vi "[RT] Finite Acq.vi"() -> ()   [LabVIEW 2025]
doc: "The finite acquisition mode tells the FPGA to acquire a certain number of samples and then terminate the acquisition. In this acquisition mode, the rwfm_ConfigTiming VI calls rwfm_BufferConfig.vi and sets the host application's data buffer size equal to the number of points in the finite acquisition."
uses:
  <vilib>/Utility/error.llb/DialogType.ctl
  <vilib>/NI/cRIO Wfm/ChannelConfig.ctl
  <vilib>/DAQmx/write.llb/DAQmx Write (Analog Wfm 1Chan NSamp).vi
  <vilib>/DAQmx/create/channels.llb/DAQmx Create Channel (AO-Voltage-Basic).vi
  <vilib>/DAQmx/configure/timing.llb/DAQmx Timing (Sample Clock).vi
  <vilib>/DAQmx/miscellaneous.llb/DAQmx Fill In Error Info.vi
  <vilib>/FPGAPlugInAG/cRIO-9045/niLvFpga_Open_cRIO-9045.vi
  <vilib>/rvi/interface/common/dynamic/niFpgaDynamicAddResources.vi
  <vilib>/NI/cRIO Wfm/AcqRead(Wfm).vi
  <vilib>/FPGAPlugInAG/Dynamic/niLvFpga_Close_Dynamic.vi
  <vilib>/rvi/interface/nirviOpenFPGA/nirviOpenFPGA.xnode
  FPGA Bitfiles/criowaveformexam_FPGATarget2_[FPGA]DeltaSigan_kh7RgRjxIrM.lvbitx
  <vilib>/rvi/interface/nirviCloseFPGA/nirviCloseFPGA.xnode
  <vilib>/NI/cRIO Wfm/cRIO Wfm.lvlib
  <resource>/objmgr/daqmx.rc
  <vilib>/measure/NI_MABase.lvlib
panel:
  out "error out":errorcluster
  out "AO Waveform Graph":waveform(dbl)(graph)
  out "Actual AO Sample Rate":dbl=1000.0 format="%0.2f"
  in  "Stop":bool
  out "Acquired Data Graph":waveform(sgl)[](graph)
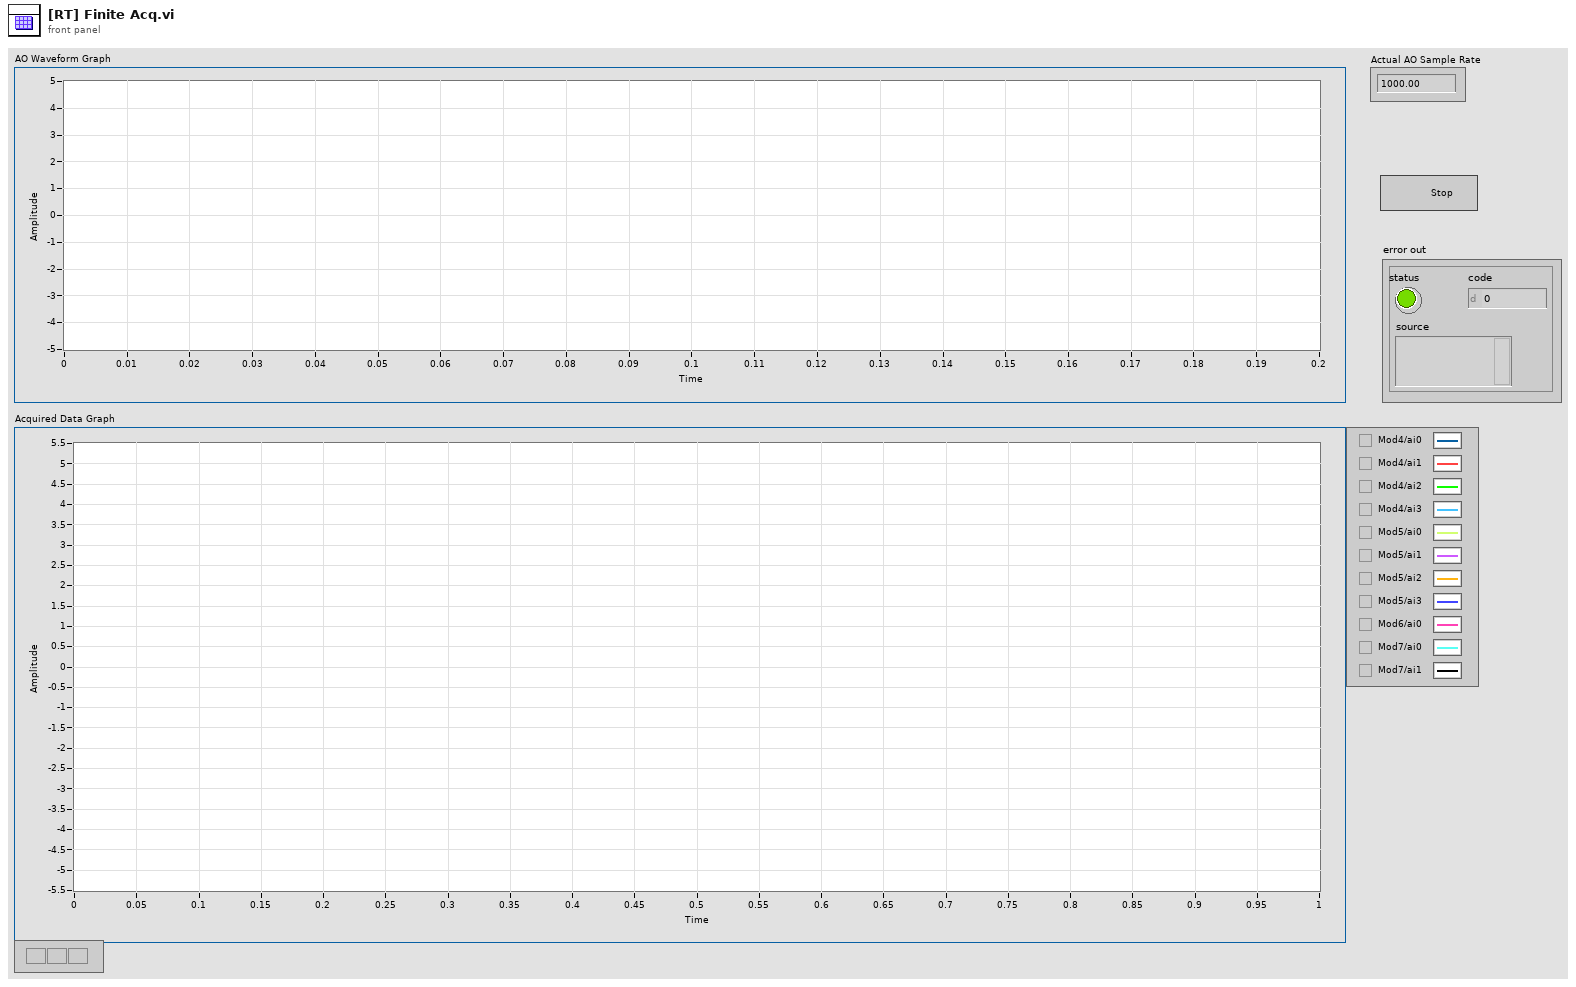
[diagram p1: front panel]
types:
  T1 = typedef "cRIO Wfm.lvlib/ChannelConfig.ctl" = cluster{"Channel Name":string, "Sensitivity mV_EU":dbl, "EU":string, "dB Ref EU":dbl}[]
  T2 = typedef "DialogType.ctl" = u16
  T3 = typedef "cRIO Wfm.lvlib/SamplingInfo.ctl" = cluster{"Number of Channels":i32, "Actual Samp Rate":dbl, "Chan Name Array":string[], "EU Chan Array":string[], "dB Ref Chan Array":dbl[]}
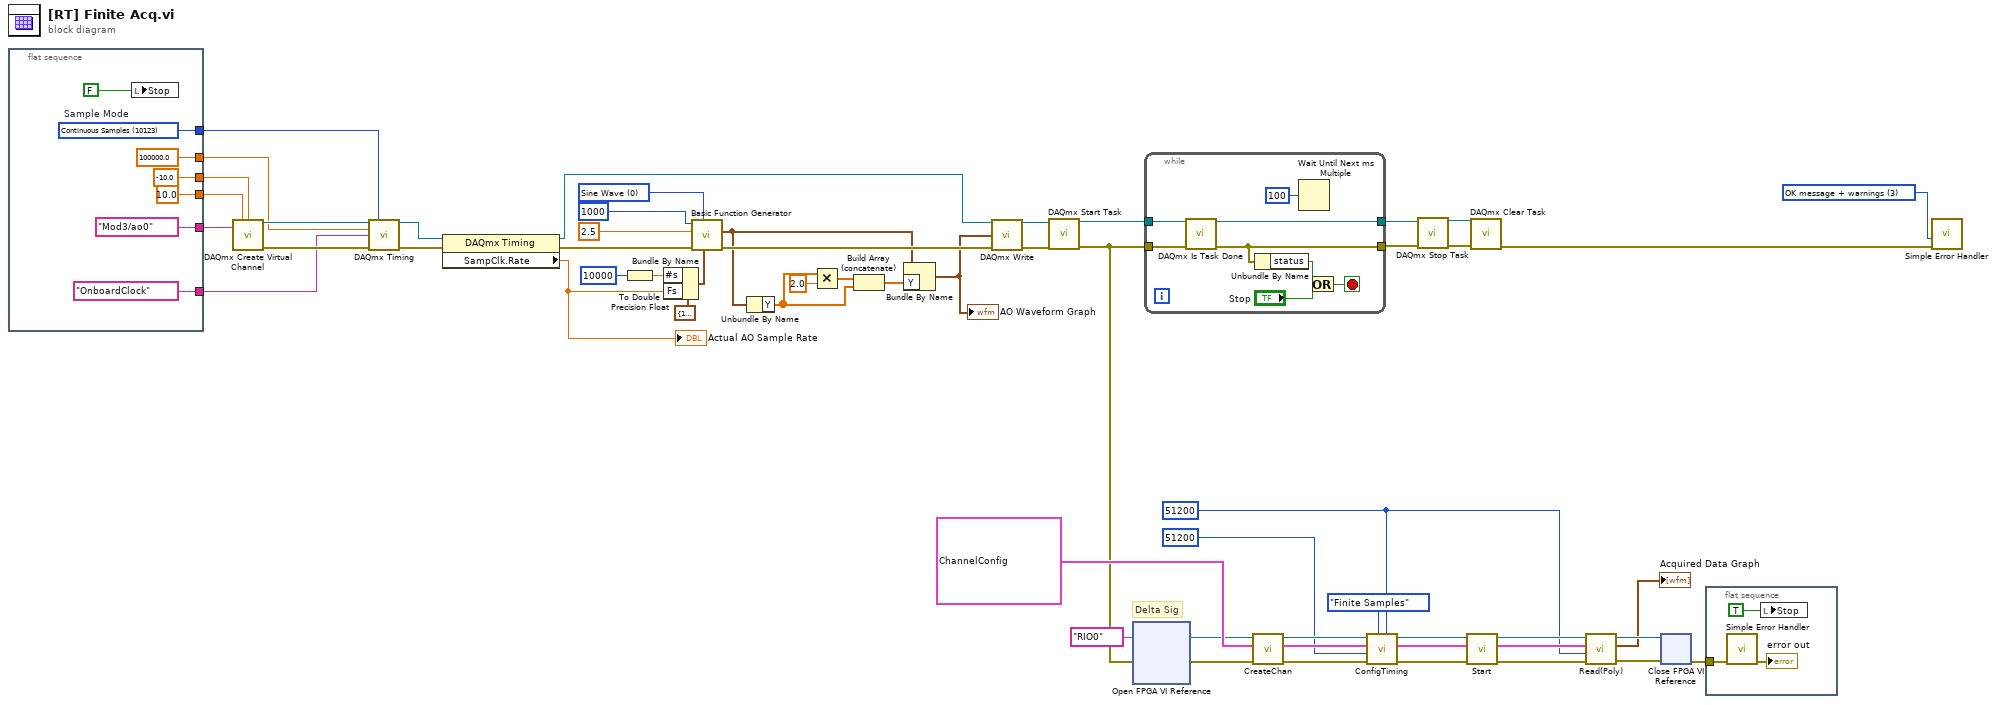
[diagram p0: block diagram]
diagram:
  w44 = 51200 ("Samps per Chan")
  w11 = u16 0 items=["Sine Wave", "Triangle Wave", "Square Wave", "Sawtooth Wave"] ("Waveform Type")
  w23 = T2 3 items=["no dialog", "OK message", "continue or stop message", "OK message + warnings", "continue/stop + warnings"] ("type of dialog (OK msg:1)")
  # "Delta Sig"
  n1 = flat-sequence {
    tunnel: [tag "Mod3/ao0" ("Pure Tone Channel")] -> w20
    tunnel: [-10.0 ("Min Voltage")] -> w19
    tunnel: [10.0 ("Max Voltage")] -> w18
    tunnel: [tag "OnboardClock" ("Sample Clock Source")] -> w17
    tunnel: [100000.0 ("Sample Rate")] -> w16
    tunnel: [w58] -> w15
    frame #0 {
      w58 = 10123 items=["Finite Samples"=10178, "Continuous Samples"=10123, "Hardware Timed Single Point"=12522]  # Sample Mode
      n2 = local write "Stop"(FALSE ("stop")) -> ()
    }
  }
  n3 = call-poly <vilib>:"DAQmx Create Virtual Channel.vi"("maximum value"=w18, "minimum value"=w19, "physical channels"=w20) -> ("task out"=w36:refnum<k21>, "error out"=w37:errorcluster)  [unwired: 11 in]
  n4 = call-poly <vilib>:"DAQmx Timing.vi"("task/channels in"=w36, "sample mode"=w15, "rate"=w16, "source"=w17, "error in"=w37) -> ("task out"=w14:refnum<k21>, "error out"=w38:errorcluster)  [unwired: 9 in]
  n5 = property class="DAQmx Timing"(reference=w14, error in=w38) -> (reference out=w21:refnum<k21>, error out=w22:errorcluster, "SampClk.Rate"=w32:dbl)
  "Actual AO Sample Rate" <- w32
  n6 = To Double Precision Float(number=10000 ("Number of Samples")) -> (double precision float=w29:dbl)
  n7 = Bundle By Name(cluster=cluster{"Fs":dbl, "#s":dbl} {"Fs"=1000.0, "#s"=1000.0} ("sampling info"), "#s"=w29, "Fs"=w32) -> (w10:cluster{"Fs":dbl, "#s":dbl})
  n8 = call <vilib>:"Basic Function Generator.vi"("sampling info"=w10, "signal type"=w11, "error in (no error)"=w22, "amplitude"=2.5 ("Amplitude"), "frequency"=1000 ("Frequency")) -> ("error out"=w9:errorcluster, "signal out"=w5:waveform(dbl))  [unwired: 4 in, 1 out]
  n9 = Unbundle By Name(w5) -> ("Y"=w8:dbl[])
  n10 = Multiply(x=w8, y=2.0) -> (x*y=w6:dbl[])
  n11 = Build Array (concatenate)(w6, w8) -> (w4:dbl[])
  n12 = Bundle By Name(cluster=w5, "Y"=w4) -> (w3:waveform(dbl))
  "AO Waveform Graph" <- w3
  n13 = call-poly <vilib>:"DAQmx Write.vi"("task/channels in"=w21, "data"=w3, "error in"=w9) -> ("task out"=w31:refnum<k21>, "error out"=w30:errorcluster)  [unwired: 10 in, 1 out]
  n14 = call <vilib>:"DAQmx Start Task.vi"("task/channels in"=w31, "error in"=w30) -> ("task out"=w35:refnum<k21>, "error out"=w2:errorcluster)  [unwired: 12 in]
  n15 = xnode "Open FPGA VI Reference"("error in"=w2, "resource name"=tag "RIO0") -> ("FPGA VI Reference Out"=w40:refnum<k20>, "error out"=w39:errorcluster)
  n16 = while {
    tunnel: w35 -> [w72]
    tunnel: w2 -> [w71]
    tunnel: [w68] -> w24
    tunnel: [w69] -> w25
    stop <- w70 stop-if-true
    n17 = call <vilib>:"DAQmx Is Task Done.vi"("task/channels in"=w72, "error in"=w71) -> ("task out"=w69:refnum<k21>, "error out"=w68:errorcluster)  [unwired: 11 in, 1 out]
    n18 = Unbundle By Name(w68) -> ("status"=w67:bool)
    n19 = Wait Until Next ms Multiple(millisecond multiple=u32 100) -> ()  [unwired: 1 out]
    n20 = Or(x=w67, y="Stop") -> (x .or. y?=w70:bool)
  }
  n21 = call <vilib>:"CreateChan.vi"("error in"=w39, "Channel Info"=T1 [{"Channel Name"="Mod4/ai0", "Sensitivity mV_EU"=1000.0, "EU"="V", "dB Ref EU"=1.0}, {"Channel Name"="Mod4/ai1", "Sensitivity mV_EU"=1000.0, "EU"="V", "dB Ref EU"=1.0}, {"Channel Name"="Mod4/ai2", "Sensitivity mV_EU"=1000.0, "EU"="V", "dB Ref EU"=1.0}, {"Channel Name"="Mod4/ai3", "Sensitivity mV_EU"=1000.0, "EU"="V", "dB Ref EU"=1.0}, {"Channel Name"="Mod5/ai0", "Sensitivity mV_EU"=1000.0, "EU"="V", "dB Ref EU"=1.0}, {"Channel Name"="Mod5/ai1", "Sensitivity mV_EU"=1000.0, "EU"="V", "dB Ref EU"=1.0}, {"Channel Name"="Mod5/ai2", "Sensitivity mV_EU"=1000.0, "EU"="V", "dB Ref EU"=1.0}, {"Channel Name"="Mod5/ai3", "Sensitivity mV_EU"=1000.0, "EU"="V", "dB Ref EU"=1.0}, {"Channel Name"="Mod6/ai0", "Sensitivity mV_EU"=1000.0, "EU"="V", "dB Ref EU"=1.0}, {"Channel Name"="Mod7/ai0", "Sensitivity mV_EU"=1000.0, "EU"="V", "dB Ref EU"=1.0}, {"Channel Name"="Mod7/ai1", "Sensitivity mV_EU"=1000.0, "EU"="V", "dB Ref EU"=1.0}], "Dynamic FPGA Ref"=w40) -> ("error out"=w54:errorcluster, "Sampling Info"=w53:T3, "Dynamic FPGA Ref Out"=w55:refnum<k20>)  [unwired: 1 in, 5 out]
  n22 = call <vilib>:"ConfigTiming.vi"("Samples per Channel"=w44, "Sample Mode"=enum16{"Finite Samples", "Continuous Samples"}."Finite Samples", "error in"=w54, "Sample Rate"=u32 51200, "Sampling Info In"=w53, "Dynamic FPGA Ref"=w55) -> ("error out"=w47:errorcluster, "Sampling Info Out"=w48:T3, "Dynamic FPGA Ref Out"=w49:refnum<k20>)  [unwired: 2 in, 1 out]
  n23 = call <vilib>:"DAQmx Stop Task.vi"("task/channels in"=w25, "error in"=w24) -> ("task out"=w27:refnum<k21>, "error out"=w26:errorcluster)  [unwired: 12 in]
  n24 = call <vilib>:"Start.vi"("error in"=w47, "Sampling Info In"=w48, "Dynamic FPGA Ref"=w49) -> ("error out"=w51:errorcluster, "Sampling Info Out"=w52:T3, "Dynamic FPGA Ref Out"=w50:refnum<k20>)  [unwired: 6 out]
  n25 = call <vilib>:"DAQmx Clear Task.vi"("task in"=w27, "error in"=w26) -> ("error out"=w34:errorcluster)  [unwired: 13 in]
  n26 = call-poly <vilib>:"Read(Poly).vi"("error in"=w51, "Samps Read per Chan"=w44, "Sampling Info"=w52, "Dynamic FPGA Ref"=w50) -> ("error out"=w45:errorcluster, "Wfm Data"=→"Acquired Data Graph":waveform(sgl)[], "Dynamic FPGA Ref Out"=w46:refnum<k20>)  [unwired: 2 in, 3 out]
  n27 = xnode "Close FPGA VI Reference"("FPGA VI Reference In"=w46, "error in"=w45) -> ("error out"=w56:errorcluster)
  n28 = flat-sequence {
    tunnel: w56 -> [w75]
    frame #0 {
      n29 = call <vilib>:"Simple Error Handler.vi"("error in (no error)"=w75) -> ("error out"=→"error out":errorcluster)  [unwired: 1 in, 7 out]
      n30 = local write "Stop"(TRUE ("stop")) -> ()
    }
  }
  n31 = call <vilib>:"Simple Error Handler.vi"("type of dialog (OK msg:1)"=w23, "error in (no error)"=w34) -> ()  [unwired: 3 in, 5 out]
